vi "Open File.vi"(8 "error in":errorcluster, 11 "File in":refnum<class "File.lvclass">) -> (0 "error out":errorcluster, 3 "File out":refnum<class "File.lvclass">)   [LabVIEW 2019, in "ManejoArchivos.lvlib" / "File.lvclass"]
uses:
  File.lvclass
  File.lvclass/File.ctl
  <vilib>/Utility/sysdir.llb/System Directory Type.ctl
  Write File Path.vi
  Read File Path.vi
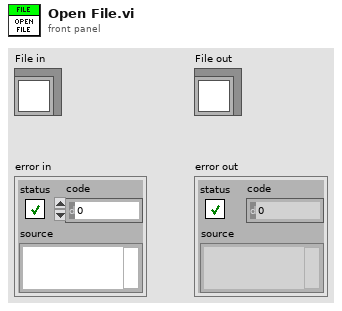
[diagram p1: front panel]
types:
  T1 = typedef "System Directory Type.ctl" = i32
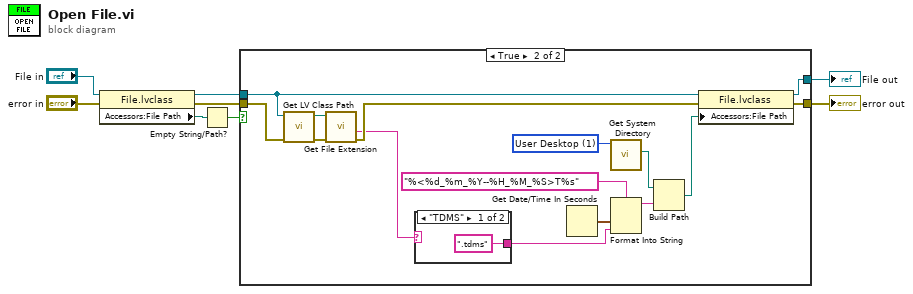
[diagram p0: block diagram]
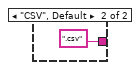
[diagram p3: hidden frame]
diagram:
  n1 = property class="File.lvclass"(reference="File in", error in="error in") -> (reference out=w2:refnum<class "File.lvclass">, error out=w6:errorcluster, "Accessors:File Path"=w4:path)
  n2 = Empty String/Path?(string/path=w4) -> (empty?=w1:bool)
  n3 = case shown="True" w1 {
    tunnel: [w10 w25] -> w7
    tunnel: w6 -> [w10 w24]
    tunnel: [w9 w21] -> w3
    tunnel: w2 -> [w9 w20]
    frame False {
    }
    frame True {
      w17 = T1 1 items=["User Home"=0, "User Desktop"=1, "User Documents"=2, "User Application Data"=3, "User Preferences"=4, "User Temporary"=5, "Public Documents"=6, "Public Application Data"=7, "Public Preferences"=8, "Public Cache"=13, "System Core Libraries"=9, "System Installed Libraries"=10, "Application Files"=11, "Boot Volume Root"=12] ("system directory type")
      n4 = call <vilib>:"Get LV Class Path.vi"("error in (no error)"=w24, "object"=w20) -> ("error out"=w23:errorcluster, "class path"=w19:path)  [unwired: 8 in]
      n5 = call <vilib>:"Get File Extension.vi"("error in (no error)"=w23, "file"=w19) -> ("error out"=w22:errorcluster, "filename without extension"=w18:string)  [unwired: 5 in, 3 out]
      n6 = case shown="\"TDMS\"" w18 {
        tunnel: [".tdms" ".csv"] -> w13
        frame "TDMS" {
        }
        frame "CSV", Default {
        }
      }
      n7 = Get Date/Time In Seconds() -> (seconds since 1Jan1904=w14:timestamp)
      n8 = call <vilib>:"Get System Directory.vi"("system directory type"=w17) -> ("system directory"=w16:path)  [unwired: 10 in]
      n9 = Format Into String(format string="%<%d_%m_%Y--%H_%M_%S>T%s", w14, w13) -> (resulting string=w12:string)  [unwired: 2 in, 1 out]
      n10 = Build Path(base path=w16, name or relative path=w12) -> (appended path=w15:path)
      n11 = property class="File.lvclass"(reference=w20, error in=w22, "Accessors:File Path"=w15) -> (reference out=w21:refnum<class "File.lvclass">, error out=w25:errorcluster)
    }
  }
  "error out" <- w7
  "File out" <- w3
